vi "quydaocoban1.vi"(9 "t":dbl, 10 "v":dbl, 11 "S0":dbl) -> (2 "S":dbl)   [LabVIEW 2019]
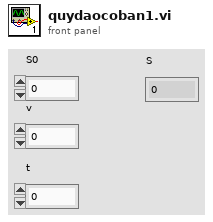
[diagram p1: front panel]
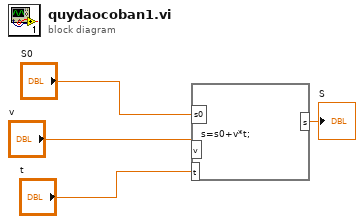
[diagram p0: block diagram]
diagram:
  n1 = formula code="s=s0+v*t;"("s0"="S0", "v"="v", "t"="t") -> ("s"=→"S":dbl)
